vi "TestLocalize.vi"() -> ()   [LabVIEW 2011]
uses:
  JelmersTracker.llb/TrackerDLL.vi
panel:
  in  "XCorWindow":u32=128
  out "max Y pos":i32
  out "max X pos":i32
  in  "Path":path
  in  "Browse?":bool
  out "Radial profile":sgl[](graph)
  in  "xcor_iterations":i32=1
  out "X autocor":sgl[](graph)
  out "Y autocor":sgl[](graph)
  out "Y profile":sgl[](graph)
  out "X profile":sgl[](graph)
  in  "debug library":bool
  out "debug":T1(plugin-control)
  out "median":sgl
  out "xcorpos":cluster{"XCor X":sgl, "XCor Y":sgl}
  out "COM":cluster{"comX":sgl, "comY":sgl}
  out "Image":T1(plugin-control)
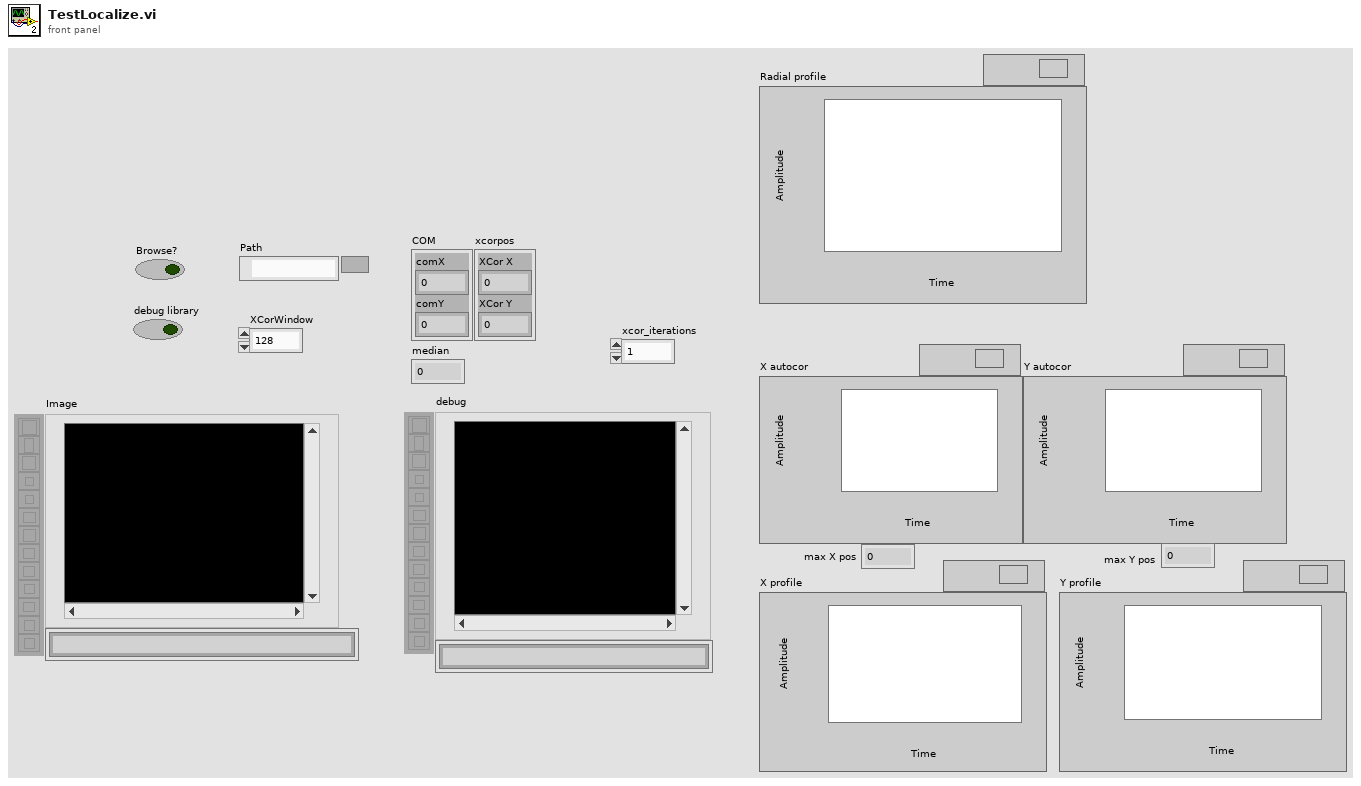
[diagram p1: front panel]
types:
  T1 = typedef "IMAQ Image.ctl" = refnum<image>
  T2 = typedef "Image Type" = u32
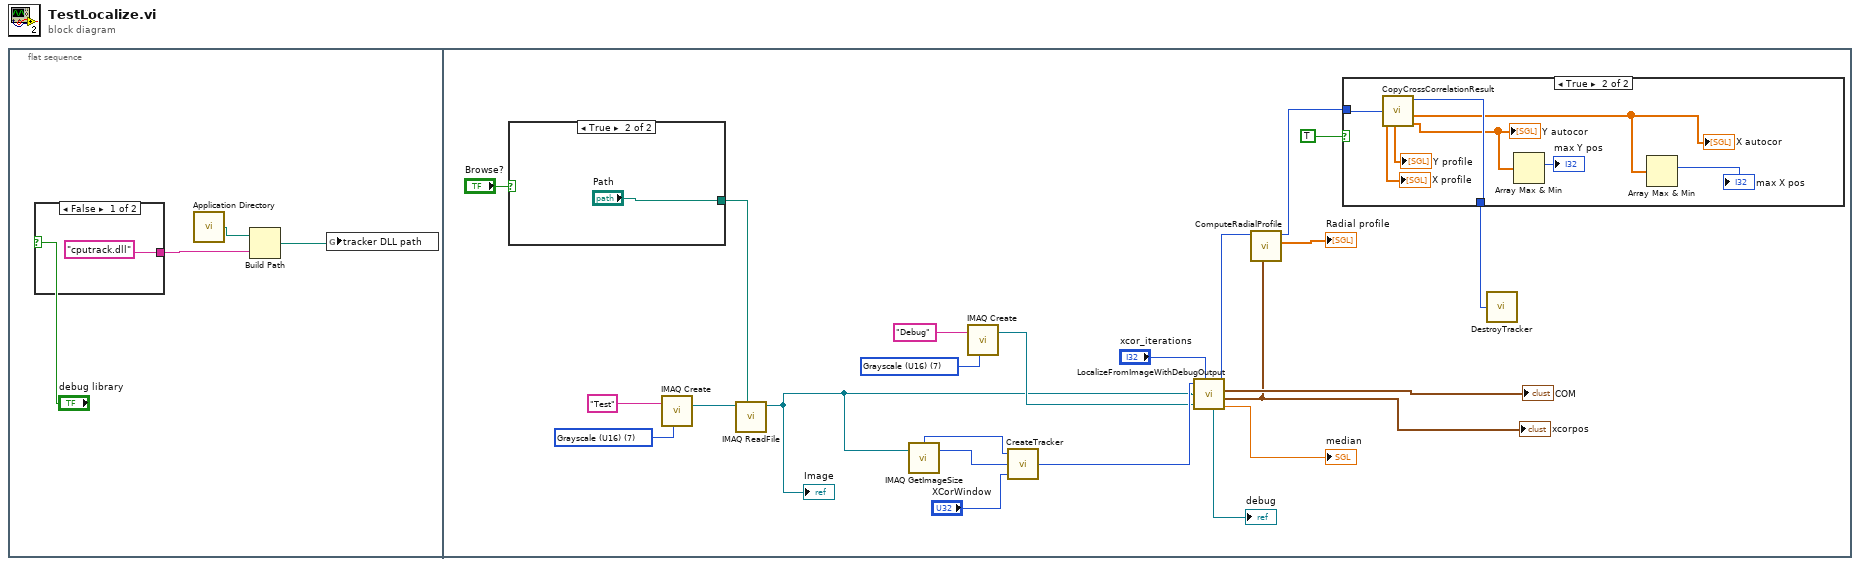
[diagram p0: block diagram]
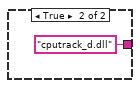
[diagram p2: hidden frame]
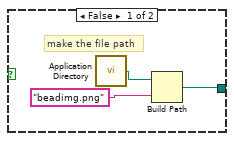
[diagram p3: hidden frame]
diagram:
  n1 = flat-sequence {
    frame #0 {
      n2 = case shown="False" "debug library" {
        tunnel: ["cputrack.dll" "cputrack_d.dll"] -> w3
        frame False {
        }
        frame True {
        }
      }
      n3 = call <vilib>:"Application Directory.vi"() -> ("Application Directory"=w2:path)
      n4 = Build Path(base path=w2, name or relative path=w3) -> (appended path=w4:path)
      n5 = global write "TrackerDLL.vi" "tracker DLL path"(w4) -> ()
    }
    frame #1 {
      w24 = T2 7 items=["Grayscale (U8)", "Grayscale (I16)", "Grayscale (SGL)", "Complex (CSG)", "RGB (U32)", "HSL (U32)", "RGB (U64)", "Grayscale (U16)"] ("Image Type")
      w26 = T2 7 items=["Grayscale (U8)", "Grayscale (I16)", "Grayscale (SGL)", "Complex (CSG)", "RGB (U32)", "HSL (U32)", "RGB (U64)", "Grayscale (U16)"] ("Image Type")
      n6 = case shown="True" "Browse?" {
        tunnel: [w30 "Path"] -> w27
        frame False {
          # "make the file path"
          n7 = call <vilib>:"Application Directory.vi"() -> ("Application Directory"=w31:path)
          n8 = Build Path(base path=w31, name or relative path="beadimg.png") -> (appended path=w30:path)
        }
        frame True {
        }
      }
      n9 = call "IMAQ Create"("Image Name"="Test" ("String"), "Image Type"=w26) -> ("New Image"=w28:T1)  [unwired: 3 in, 1 out]
      n10 = call "IMAQ ReadFile"("File Path"=w27, "Image"=w28) -> ("Image Out"=w18:T1)  [unwired: 5 in, 4 out]
      "Image" <- w18
      n11 = call "IMAQ GetImageSize"("Image"=w18) -> ("Y Resolution"=w16:i32, "X Resolution"=w17:i32)  [unwired: 3 in, 1 out]
      n12 = call "IMAQ Create"("Image Name"="Debug" ("String"), "Image Type"=w24) -> ("New Image"=w19:T1)  [unwired: 3 in, 1 out]
      n13 = call "CreateTracker.vi"("XCorWindow"="XCorWindow", "height"=w16, "width"=w17) -> ("return type"=w23:u64)
      n14 = call "LocalizeFromImageWithDebugOutput.vi"("tracker"=w23, "xcor_iterations"="xcor_iterations", "input image"=w18, "debug image"=w19) -> ("tracker"=w12:u64, "COM"=→"COM":cluster{"X":sgl, "Y":sgl}, "debug image"=→"debug":T1, "xcorpos"=w9:cluster{"X":sgl, " Y":sgl}, "median"=→"median":sgl)  [unwired: 2 in]
      "xcorpos" <- w9
      n15 = call "ComputeRadialProfile.vi"("center"=w9, "tracker"=w12) -> ("output"=→"Radial profile":sgl[], "tracker"=w11:u64)  [unwired: 8 in]
      n16 = case shown="True" TRUE {
        tunnel: w11 -> [w34 w39]
        tunnel: [w34 w42] -> w15
        frame False {
        }
        frame True {
          n17 = call "CopyCrossCorrelationResult.vi"("tracker"=w39) -> ("x prof"=→"X profile":sgl[], "y prof"=→"Y profile":sgl[], "tracker"=w42:u64, "x result"=w38:sgl[], "y_result"=w37:sgl[])  [unwired: 3 in]
          "X autocor" <- w38
          "Y autocor" <- w37
          n18 = Array Max & Min(array=w37) -> (max index (indices)=→"max Y pos":i32)  [unwired: 3 out]
          n19 = Array Max & Min(array=w38) -> (max index (indices)=→"max X pos":i32)  [unwired: 3 out]
        }
      }
      n20 = call "DestroyTracker.vi"("tracker"=w15) -> ()
    }
  }
